vi "Send JSON Path_ZA.vi"(7 "Message Priority (Normal)":T2=enum."Normal", 8 "error in (no error)":errorcluster, 10 "JSON Path":T1, 11 "Message Enqueuer":refnum<class "Message Enqueuer.lvclass">) -> (0 "error out":errorcluster, 3 "Message Enqueuer out":refnum<class "Message Enqueuer.lvclass">)   [LabVIEW 2015, in "JSON Path_ZA Msg.lvclass"]
doc: "This VI sends the message to an actor."
uses:
  JSON Path_ZA Msg.lvclass
  <vilib>/ActorFramework/Message Enqueuer/Message Enqueuer.lvclass
  <vilib>/ActorFramework/Message Enqueuer/Message Priority.ctl
  Zen Analytics/Dependency/OverWrite JSON Cluster.ctl
  JSON Path_ZA Msg.lvclass/JSON Path_ZA Msg.ctl
  <vilib>/ActorFramework/Message Enqueuer/Message Enqueuer.lvclass/Message Enqueuer.ctl
  <vilib>/ActorFramework/Message Priority Queue/Priority Enqueue.vi
  Zen Analytics/Zen Analytics.lvclass
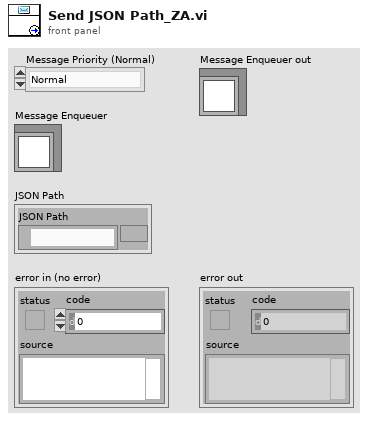
[diagram p1: front panel]
types:
  T1 = typedef "Zen Analytics.lvclass/OverWrite JSON Cluster.ctl" = cluster{"JSON Path":path}
  T2 = typedef "Actor Framework.lvlib/Message Enqueuer.lvclass/Message Priority.ctl" = enum16{"Low", "Normal", "High"}
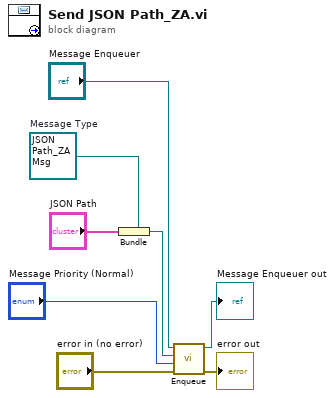
[diagram p0: block diagram]
diagram:
  w5 = refnum<class "JSON Path_ZA Msg.lvclass"> refnum  # Message Type
  n1 = Bundle(cluster=w5, "JSON Path") -> (w4:refnum<class "JSON Path_ZA Msg.lvclass">)
  n2 = call <vilib>:"Enqueue.vi"("error in (no error)"="error in (no error)", "Message Priority (Normal)"="Message Priority (Normal)", "Message"=w4, "Message Enqueuer in"="Message Enqueuer") -> ("error out"=→"error out":errorcluster, "Message Enqueuer out"=→"Message Enqueuer out":refnum<class "Message Enqueuer.lvclass">)  [unwired: 6 in]
